vi "DevID last 6bit.vi"(4 "Devid":string) -> (1 "结果字符串":string)   [LabVIEW 2013]
panel:
  out "子字符串":string
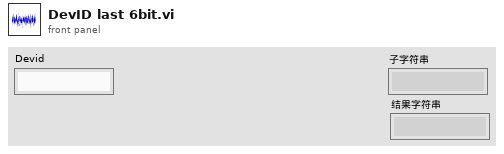
[diagram p1: front panel]
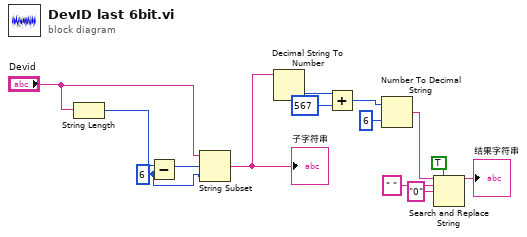
[diagram p0: block diagram]
diagram:
  w11 = 6 ("y")
  n1 = String Length(string="Devid") -> (length=w13:i32)
  n2 = Subtract(x=w13, y=w11) -> (x-y=w14:i32)
  n3 = String Subset(string="Devid", offset (0)=w14, length (rest)=w11) -> (substring=w10:string)
  "子字符串" <- w10
  n4 = Decimal String To Number(string=w10) -> (number=w9:i32)  [unwired: 2 in, 1 out]
  n5 = Add(x=w9, y=567) -> (x+y=w7:i32)
  n6 = Number To Decimal String(number=w7, width (-)=i16 6 ("宽度(-)")) -> (decimal integer string=w5:string)
  n7 = Search and Replace String(replace all?=TRUE ("替换全部？(F)"), input string=w5, search string=" " ("十进制整型字符串"), replace string="0" ("替换字符串(\"\")")) -> (result string=→"结果字符串":string)  [unwired: 4 in, 3 out]
